vi "_Main.vi"   [LabVIEW 2017, in "Arm.lvlib"]
uses:
  Arm.lvlib
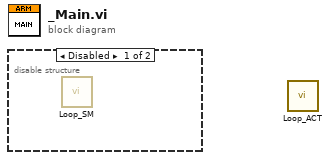
[diagram p0: block diagram]
diagram:
  n1 = disable-structure shown="Disabled" {
    frame Disabled {
      n2 = call "Loop_SM.vi"() -> ()  [unwired: 12 in]
    }
    frame Enabled {
    }
  }
  n3 = call "Loop_ACT.vi"() -> ()  [unwired: 12 in]
